vi "Read HW Angle.vi"(6 "error in":errorcluster, 8 "DATA[4-7]":u8[](array[numeric])=[124, 161, 190, 254] format="%.0x", 9 "Channel in":u16) -> (0 "error out":errorcluster, 1 "Messages":T1(array[cluster]), 2 "Pass":bool, 3 "Channel out":u16)   [LabVIEW 2023]
uses:
  7ad73885-74d4-4865-958d-ac69876d8a76.vi
  Communication/PCAN2023/PCAN API.lvlib
panel:
  out "Numeric":i32
  in  "stop 1":bool
  out "MessageBuffer out":T2 {"ID" format="%.0x"; "DATA[0]" format="%.0x"; "DATA[1]" format="%.0x"; "DATA[2]" format="%.0x"; "DATA[3]" format="%.0x"; "DATA[4]" format="%.0x"; "DATA[5]" format="%.0x"; "DATA[6]" format="%.0x"; "DATA[7]" format="%.0x"}
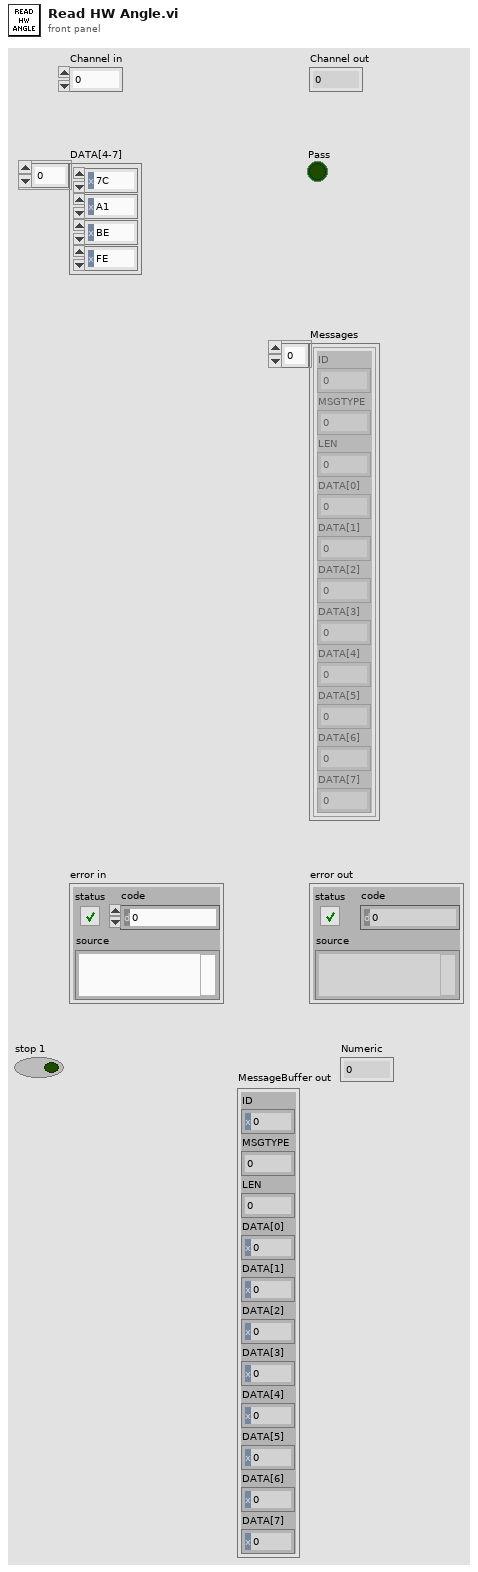
[diagram p1: front panel]
types:
  T1 = cluster{"ID":u32, "MSGTYPE":u8, "LEN":u8, "DATA[0]":u8, "DATA[1]":u8, "DATA[2]":u8, "DATA[3]":u8, "DATA[4]":u8, "DATA[5]":u8, "DATA[6]":u8, "DATA[7]":u8}[]
  T2 = cluster{"ID":u32, "MSGTYPE":u8, "LEN":u8, "DATA[0]":u8, "DATA[1]":u8, "DATA[2]":u8, "DATA[3]":u8, "DATA[4]":u8, "DATA[5]":u8, "DATA[6]":u8, "DATA[7]":u8}
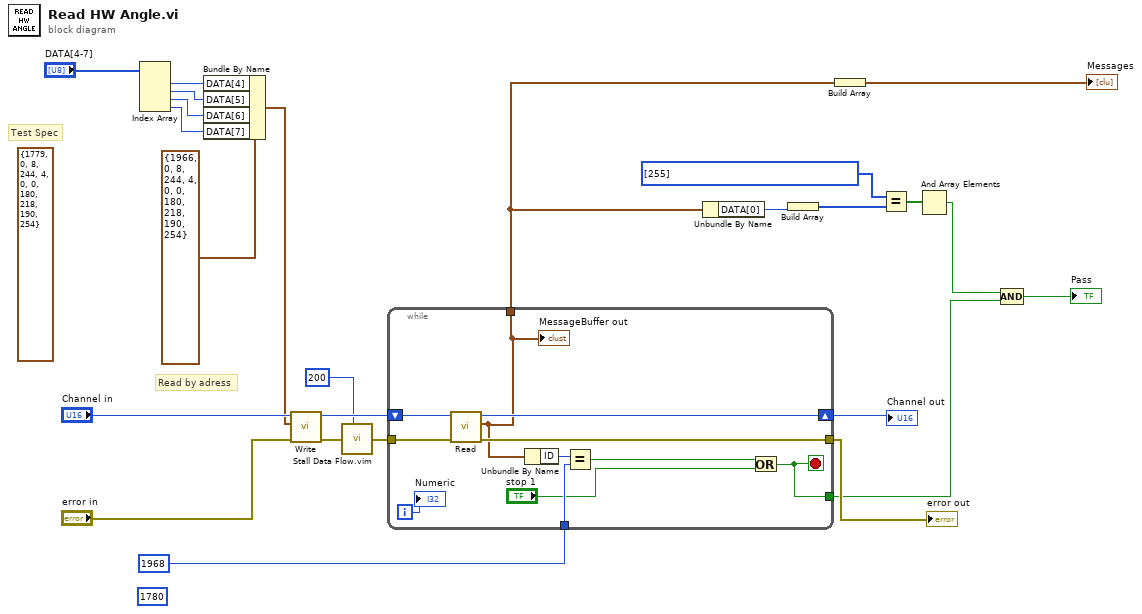
[diagram p0: block diagram]
diagram:
  (unwired) T2 {"ID"=1779, "MSGTYPE"=0, "LEN"=8, "DATA[0]"=244, "DATA[1]"=4, "DATA[2]"=0, "DATA[3]"=0, "DATA[4]"=180, "DATA[5]"=218, "DATA[6]"=190, "DATA[7]"=254} ("MessageBuffer")
  (unwired) u32 1780 ("ID")
  # "Read by adress"
  # "Test Spec"
  n1 = Index Array(array="DATA[4-7]") -> (element #1=w6:u8, element #2=w5:u8, element #3=w4:u8, element #4=w3:u8)  [unwired: 4 in]
  n2 = Bundle By Name(cluster=T2 {"ID"=1966, "MSGTYPE"=0, "LEN"=8, "DATA[0]"=244, "DATA[1]"=4, "DATA[2]"=0, "DATA[3]"=0, "DATA[4]"=180, "DATA[5]"=218, "DATA[6]"=190, "DATA[7]"=254} ("MessageBuffer"), "DATA[4]"=w6, "DATA[5]"=w5, "DATA[6]"=w4, "DATA[7]"=w3) -> (w9:T2)
  n3 = call "Write.vi"("error in"="error in", "MessageBuffer"=w9, "Channel"="Channel in") -> ("error out"=w24:errorcluster, "Channel out"=w23:u16)  [unwired: 5 in, 2 out]
  n4 = call "Stall Data Flow.vim"("value in"=w24, "milliseconds to wait"=u32 200) -> ("value out"=w15:errorcluster)  [unwired: 1 out]
  n5 = while {
    shift-right: [w34] -> w20
    shift-left: w23 -> [w35]
    tunnel: u32 1968 ("ID") -> [w31]
    tunnel: [w27] -> w13
    tunnel: [w28] -> w17
    tunnel: w15 -> [w36]
    tunnel: [w33] -> w19
    i -> [w30]
    stop <- w28 stop-if-true
    n6 = call "Read.vi"("error in"=w36, "Channel"=w35) -> ("error out"=w33:errorcluster, "MessageBuffer out"=w27:T2, "Channel out"=w34:u16)  [unwired: 6 in, 1 out]
    "MessageBuffer out" <- w27
    n7 = Unbundle By Name(w27) -> ("ID"=w32:u32)
    n8 = Equal?(x=w32, y=w31) -> (x = y?=w26:bool)
    n9 = Or(x=w26, y="stop 1") -> (x .or. y?=w28:bool)
    "Numeric" <- w30
  }
  "error out" <- w19
  "Channel out" <- w20
  n10 = Unbundle By Name(w13) -> ("DATA[0]"=w2:u8)
  n11 = Build Array(w2) -> (w1:u8[])
  n12 = Build Array(w13) -> (→"Messages":T1)
  n13 = Equal?(x=u8[] [255], y=w1) -> (x = y?=w11:bool[])
  n14 = And Array Elements(Boolean array=w11) -> (logical AND=w10:bool)
  n15 = Compound Arithmetic op=AND(w10, w17) -> (→"Pass":bool)
